vi "C64_scheduler.vi"(9 "periods":u32[](array[numeric])=[10000, 200, 10000], 10 "next time in":u32[](array[numeric]), 11 "global clock":u32) -> (2 "next time out":u32[](array[numeric]), 3 "chip":u8)   [LabVIEW 2018]
panel:
  in  "chip":u8[](array[numeric])=[1, 3, 255]
  # "chip code\n1 = CIA_1\n2 = CIA_2\n3 = VIC\n..\n255 = GUI"
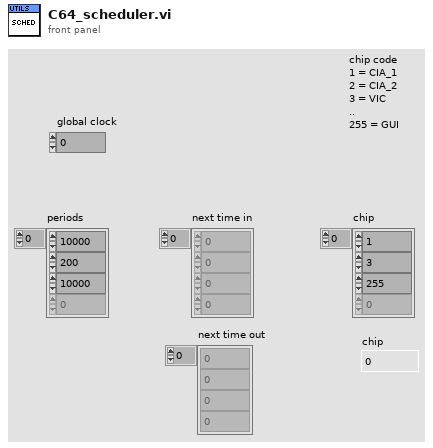
[diagram p1: front panel]
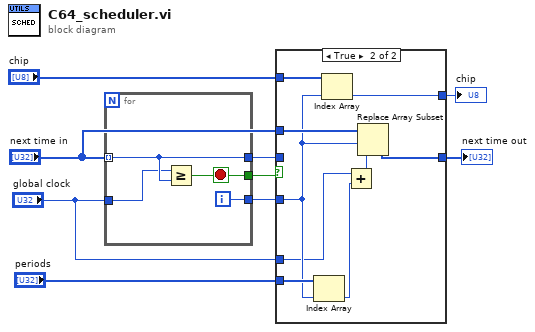
[diagram p0: block diagram]
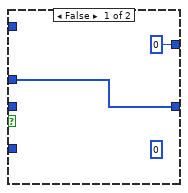
[diagram p2: hidden frame]
diagram:
  n1 = for {
    tunnel: "next time in" -> [w11] mode=indexing
    tunnel: "global clock" -> [w10]
    tunnel: [w13] -> w9
    tunnel: [w12] -> w7
    tunnel: [w11] -> w5
    i -> [w12]
    stop <- w13 stop-if-true
    n2 = Greater Or Equal?(x=w10, y=w11) -> (x >= y?=w13:bool)
  }
  n3 = case shown="True" w9 {
    tunnel: "chip" -> [_ w24]
    tunnel: w7 -> [_ w19]
    tunnel: [u8 0 ("Numeric") w23] -> w2
    tunnel: "periods" -> [_ w22]
    tunnel: w5 -> [_ _]
    tunnel: [w15 w20] -> w4
    tunnel: "next time in" -> [w15 w21]
    tunnel: "global clock" -> [_ w16]
    frame False {
      (unwired) u32 0 ("Numeric")
    }
    frame True {
      n4 = Index Array(array=w22, index=w19) -> (element=w17:u32)
      n5 = Index Array(array=w24, index=w19) -> (element=w23:u8)
      n6 = Add(x=w16, y=w17) -> (x+y=w18:u32)
      n7 = Replace Array Subset(array=w21, new element=w18, index=w19) -> (w20:u32[])
    }
  }
  "next time out" <- w4
  "chip" <- w2
